vi "Create Optimiser Cell.vi"(8 "error in (no error)":errorcluster, 11 "Schedule Cell in":refnum<class "Schedule Cell.lvclass">) -> (0 "error out":errorcluster, 3 "Optimiser Cell out":refnum<class "Optimiser Cell.lvclass">)   [LabVIEW 2020, in "Run Utilities.lvlib" / "Optimiser Cell.lvclass"]
uses:
  Optimiser Cell.lvclass
  C:/LabVIEW Code/aegis-labview-code/CIRCUS uServices et al/Run Utilities/Cell/Schedule Cell.lvclass
  Cell/Schedule Cell.lvclass
  Run Instance/Run Instance.lvclass
  Optimiser Cell.lvclass/Optimiser Cell.ctl
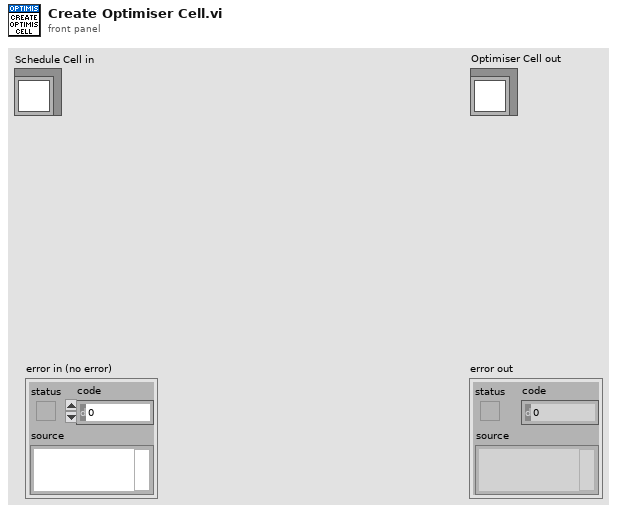
[diagram p1: front panel]
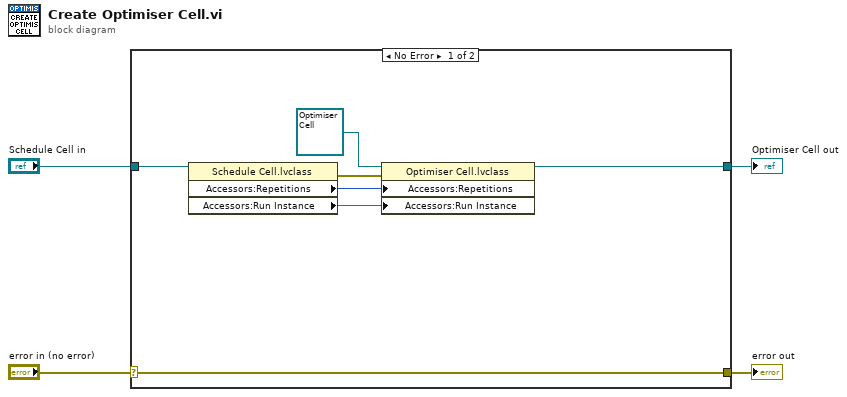
[diagram p0: block diagram]
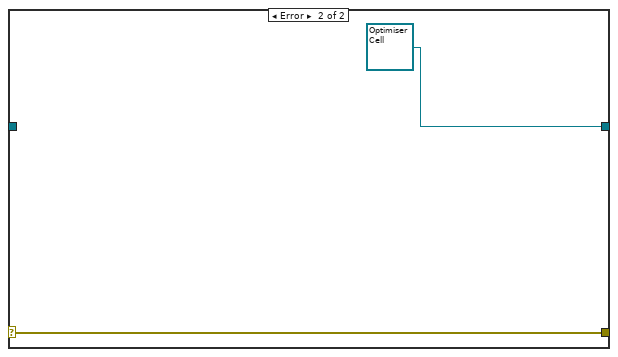
[diagram p2: hidden frame]
diagram:
  n1 = case shown="No Error" "error in (no error)" {
    selector: "error in (no error)" -> [w11 w13]
    tunnel: [w11 w13] -> w3
    tunnel: "Schedule Cell in" -> [w8 _]
    tunnel: [w9 refnum<class "Optimiser Cell.lvclass"> refnum ("Optimiser Cell out")] -> w1
    frame No Error {
      n2 = property class="Schedule Cell.lvclass"(reference=w8) -> (error out=w5:errorcluster, "Accessors:Repetitions"=w7:u32, "Accessors:Run Instance"=w6:refnum<class "Run Instance.lvclass">)  [unwired: 1 in, 1 out]
      n3 = property class="Optimiser Cell.lvclass"(reference=refnum<class "Optimiser Cell.lvclass"> refnum ("Optimiser Cell out"), error in=w5, "Accessors:Repetitions"=w7, "Accessors:Run Instance"=w6) -> (reference out=w9:refnum<class "Optimiser Cell.lvclass">)  [unwired: 1 out]
    }
    frame Error {
    }
  }
  "error out" <- w3
  "Optimiser Cell out" <- w1
